vi "Filter_Channel_Information.vi"(9 "Channel_Information_Control":T1 {"Input Terminal Configuration" items=["default"=-1, "RSE"=10083, "NRSE"=10078, "Differential"=10106, "Pseudodifferential"=12529]}) -> (1 "Array":T2[](array[typedef]) {"Input Terminal Configuration" items=["default"=-1, "RSE"=10083, "NRSE"=10078, "Differential"=10106, "Pseudodifferential"=12529]})   [LabVIEW 2021]
uses:
  typedef/Channel_Information_Control_single.ctl
  typedef/Channel_Information_Control_array.ctl
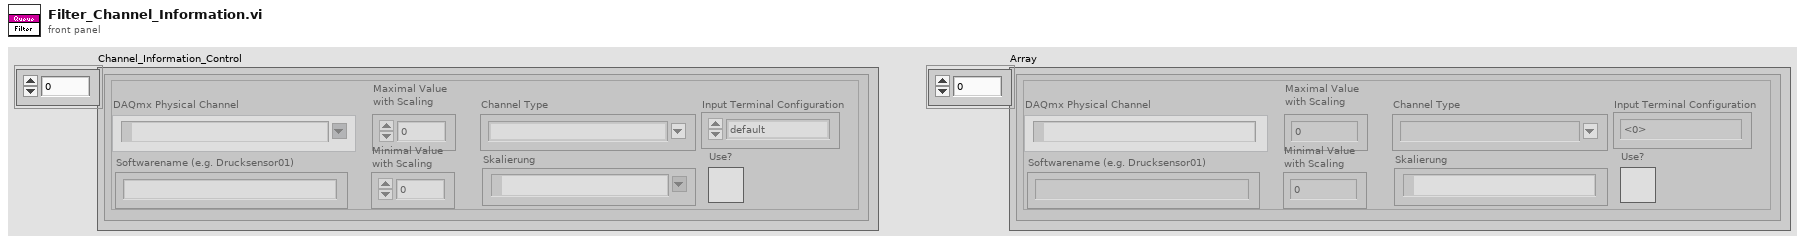
[diagram p1: front panel]
types:
  T1 = typedef "Channel_Information_Control_array.ctl" = T2[]
  T2 = typedef "Channel_Information_Control_single.ctl" = cluster{"DAQmx Physical Channel":tag, "Softwarename (e.g. Drucksensor01)":string, "Maximal Value \nwith Scaling":dbl, "Minimal Value\nwith Scaling":dbl, "Channel Type":string, "Input Terminal Configuration":i32, "Skalierung":tag, "Use?":bool}
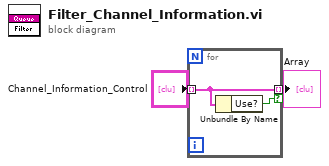
[diagram p0: block diagram]
diagram:
  n1 = for {
    tunnel: "Channel_Information_Control" -> [w4] mode=indexing
    tunnel: [w4] -> w2 mode=indexing if=w3
    n2 = Unbundle By Name(w4) -> ("Use?"=w3:bool)
  }
  "Array" <- w2
